vi "read data.vi"(8 "error in":errorcluster, 9 "timeout":i32=-1, 10 "max size":i32=10000, 11 "lvlibretls connection in":refnum<class "lvlibretls connection.lvclass">) -> (0 "error out":errorcluster, 2 "data":string, 3 "lvlibretls connection out":refnum<class "lvlibretls connection.lvclass">)   [LabVIEW 2016, in "lvlibretls connection.lvclass"]
doc: "Reads up to specified number of bytes, will usually be limited to low kb at a time."
uses:
  lvlibretls connection.lvclass
  lvlibretls connection.lvclass/lvlibretls connection.ctl
  tls library paths.vi
  lv tls dll.lvlib
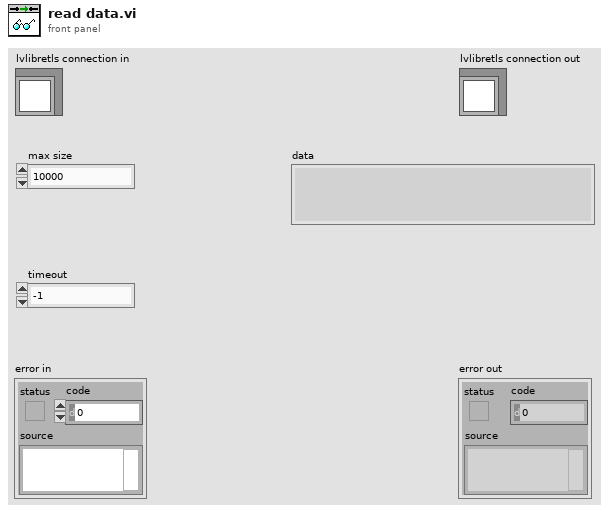
[diagram p1: front panel]
types:
  T1 = enum16{"Standard", "Buffered", "CRLF", "Immediate"}
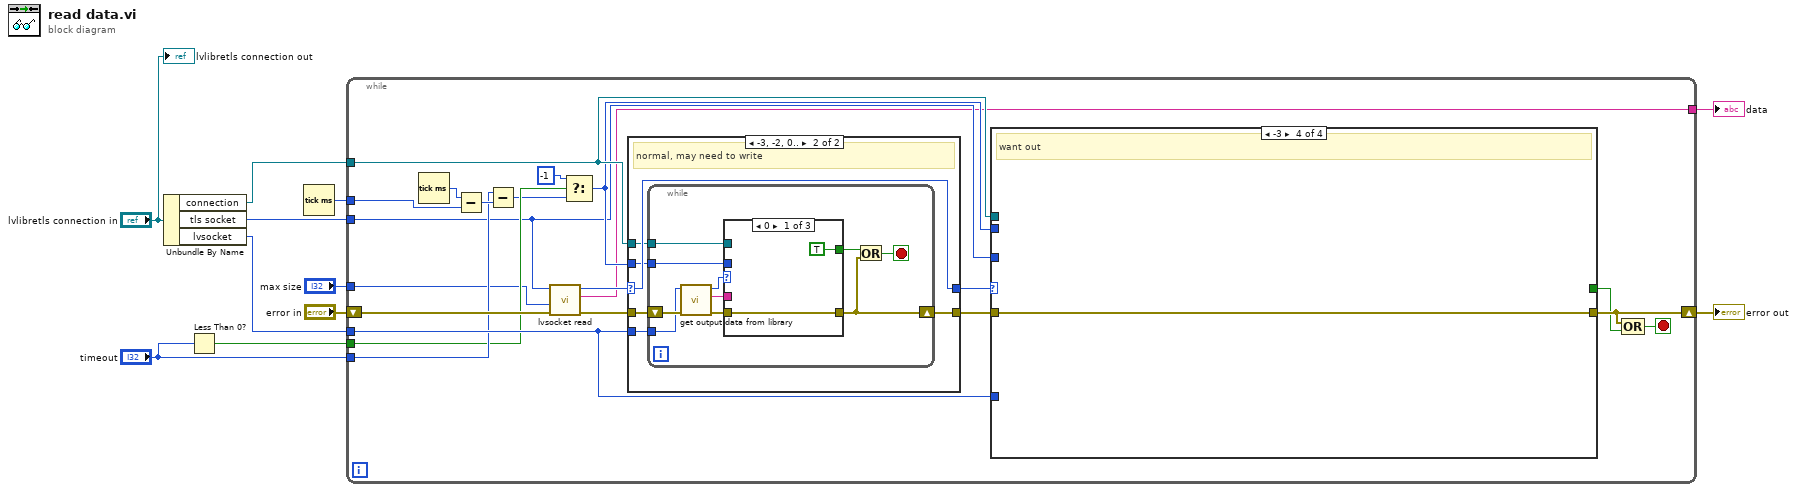
[diagram p0: block diagram]
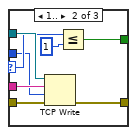
[diagram p3: hidden frame]
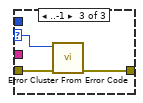
[diagram p4: hidden frame]
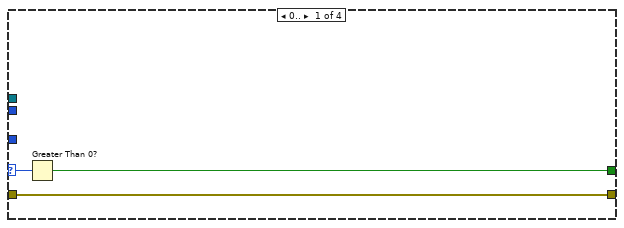
[diagram p5: hidden frame]
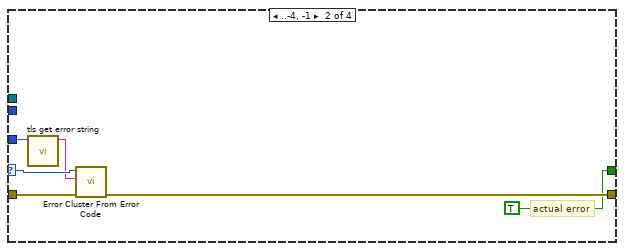
[diagram p6: hidden frame]
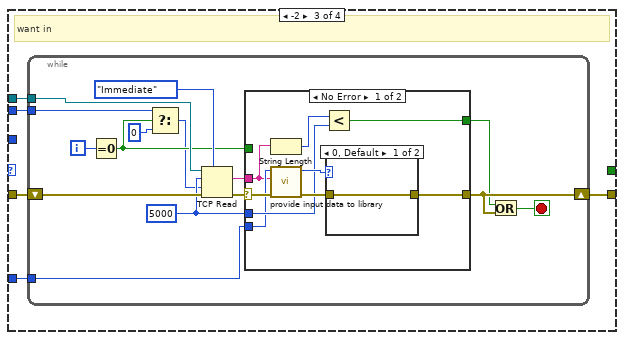
[diagram p7: hidden frame]
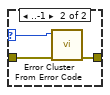
[diagram p8: hidden frame]
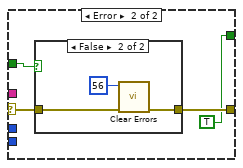
[diagram p9: hidden frame]
diagram:
  n1 = Unbundle By Name("lvlibretls connection in") -> ("connection"=w10:refnum<k5>, "tls socket"=w8:u64, "lvsocket"=w7:u64)
  n2 = Less Than 0?(x="timeout") -> (x < 0?=w6:bool)
  n3 = Tick Count (ms)() -> (millisecond timer value=w9:u32)
  n4 = while {
    shift-right: [w31] -> w3
    shift-left: "error in" -> [w32]
    tunnel: w8 -> [w14]
    tunnel: w10 -> [w23]
    tunnel: w7 -> [w24]
    tunnel: "timeout" -> [w19]
    tunnel: w6 -> [w18]
    tunnel: w9 -> [w21]
    tunnel: [w13] -> w2
    tunnel: "max size" -> [w12]
    stop <- w30 stop-if-true
    n5 = Tick Count (ms)() -> (millisecond timer value=w22:u32)
    n6 = Subtract(x=w22, y=w21) -> (x-y=w20:u32)
    n7 = Subtract(x=w19, y=w20) -> (x-y=w17:i32)
    n8 = call "lvsocket read.vi"("error in"=w32, "max read size"=w12, "tls context"=w14) -> ("error out"=w25:errorcluster, "buffer"=w13:string, "error response"=w28:i32)  [unwired: 6 in]
    n9 = Select(t=-1, s=w18, f=w17) -> (s? t:f=w15:i32)
    n10 = case shown="-3, -2, 0.." w28 {
      selector: w28 -> [w33 w40]
      tunnel: [w33 w40] -> w27
      tunnel: [w34 w38] -> w26
      tunnel: w25 -> [w34 w39]
      tunnel: w24 -> [_ w37]
      tunnel: w23 -> [_ w36]
      tunnel: w15 -> [_ w35]
      frame Default {
      }
      frame -3, -2, 0.. {
        # "normal, may need to write"
        n11 = while {
          shift-right: [w47] -> w38
          shift-left: w39 -> [w50]
          tunnel: w37 -> [w46]
          tunnel: w36 -> [w45]
          tunnel: w35 -> [w41]
          stop <- w44 stop-if-true
          n12 = call "get output data from library.vi"("error in"=w50, "lvsocket"=w46) -> ("error out"=w49:errorcluster, "data"=w42:string, "err"=w48:i32)  [unwired: 7 in]
          n13 = case shown="0" w48 {
            selector: w48 -> [_ w56 w62]
            tunnel: w49 -> [w52 w60 w63]
            tunnel: [w52 w59 w61] -> w47
            tunnel: w42 -> [_ w58 _]
            tunnel: w45 -> [_ w57 _]
            tunnel: [TRUE w54 _] -> w43
            tunnel: w41 -> [_ w53 _]
            frame 0 {
            }
            frame 1.. {
              n14 = TCP Write(connection ID=w57, data in=w58, error in (no error)=w60, 9:w53) -> (error out=w59:errorcluster)  [unwired: 2 out]
              n15 = Less Or Equal?(x=w56, y=1) -> (x <= y?=w54:bool)
            }
            frame ..-1 {
              n16 = call <vilib>:"Error Cluster From Error Code.vi"("error in (no error)"=w63, "error code (0)"=w62) -> ("error out"=w61:errorcluster)  [unwired: 7 in]
            }
          }
          n17 = Or(x=w43, y=w47) -> (x .or. y?=w44:bool)
        }
      }
    }
    n18 = case shown="-3" w27 {
      selector: w27 -> [w64 w72 _ _]
      tunnel: [w66 w71 w75 w114] -> w31
      tunnel: [w65 TRUE _ _] -> w29
      tunnel: w23 -> [_ _ w77 _]
      tunnel: w24 -> [_ _ w76 _]
      tunnel: w26 -> [w66 w69 w74 w114]
      tunnel: w15 -> [_ _ w73 _]
      tunnel: w14 -> [_ w68 _ _]
      frame 0.. {
        n19 = Greater Than 0?(x=w64) -> (x > 0?=w65:bool)
      }
      frame ..-4, -1 {
        # "actual error"
        n20 = call "tls get error string.vi"("tls context"=w68) -> ("error string"=w67:string)  [unwired: 9 in, 1 out]
        n21 = call <vilib>:"Error Cluster From Error Code.vi"("error in (no error)"=w69, "error message (\"\")"=w67, "error code (0)"=w72) -> ("error out"=w71:errorcluster)  [unwired: 6 in]
      }
      frame -2 {
        # "want in"
        n22 = while {
          tunnel: w77 -> [w92]
          tunnel: w76 -> [w89]
          shift-right: [w87] -> w75
          shift-left: w74 -> [w88]
          tunnel: w73 -> [w80]
          i -> [w86]
          stop <- w85 stop-if-true
          w83 = 5000 ("bytes to read")
          n23 = Equal To 0?(x=w86) -> (x = 0?=w81:bool)
          n24 = Select(t=w80, s=w81, f=0 ("timeout ms (25000)")) -> (s? t:f=w78:i32)
          n25 = TCP Read(connection ID=w92, bytes to read=w83, error in (no error)=w88, 7:T1."Immediate" ("mode (standard)"), 9:w78) -> (data out=w82:string, error out=w90:errorcluster)  [unwired: 1 out]
          n26 = case shown="No Error" w90 {
            selector: w90 -> [w101 w109]
            tunnel: w82 -> [w93 _]
            tunnel: w89 -> [w94 _]
            tunnel: [w98 w108] -> w87
            tunnel: w81 -> [_ w107]
            tunnel: [w95 TRUE] -> w84
            tunnel: w83 -> [w96 _]
            frame No Error {
              n27 = String Length(string=w93) -> (length=w97:i32)
              n28 = call "provide input data to library.vi"("error in"=w101, "data in"=w93, "lvsocket"=w94) -> ("error out"=w100:errorcluster, "return"=w99:i32)  [unwired: 7 in]
              n29 = Less?(x=w97, y=w96) -> (x < y?=w95:bool)
              n30 = case shown="0, Default" w99 {
                selector: w99 -> [_ w104]
                tunnel: w100 -> [w102 w105]
                tunnel: [w102 w103] -> w98
                frame 0, Default {
                }
                frame ..-1 {
                  n31 = call <vilib>:"Error Cluster From Error Code.vi"("error in (no error)"=w105, "error code (0)"=w104) -> ("error out"=w103:errorcluster)  [unwired: 7 in]
                }
              }
            }
            frame Error {
              n32 = case shown="False" w107 {
                tunnel: w109 -> [w110 w113]
                tunnel: [w110 w112] -> w108
                frame True {
                }
                frame False {
                  n33 = call <vilib>:"Clear Errors.vi"("error in (no error)"=w113, "specific error code to clear (0: all)"=56) -> ("error out"=w112:errorcluster)  [unwired: 4 in, 1 out]
                }
              }
            }
          }
          n34 = Or(x=w84, y=w87) -> (x .or. y?=w85:bool)
        }
      }
      frame -3 {
        # "want out"
      }
    }
    n35 = Compound Arithmetic op=OR(w31, w29) -> (w30:bool)
  }
  "error out" <- w3
  "data" <- w2
  "lvlibretls connection out" <- "lvlibretls connection in"
